vi "Take LTI ULS Reading.vi"(8 "error in (no error)":errorcluster, 11 "MWWL Verification in":refnum<class "MWWL Verification.lvclass">) -> (0 "error out":errorcluster, 3 "MWWL Verification out":refnum<class "MWWL Verification.lvclass">)   [LabVIEW 2017, in "MWWL Verification.lvlib" / "MWWL Verification.lvclass"]
uses:
  MWWL Verification.lvclass
  LTI ULS Actor/LTI ULS Actor Messages/Measure LTI ULS Msg/Measure LTI ULS Msg.lvclass
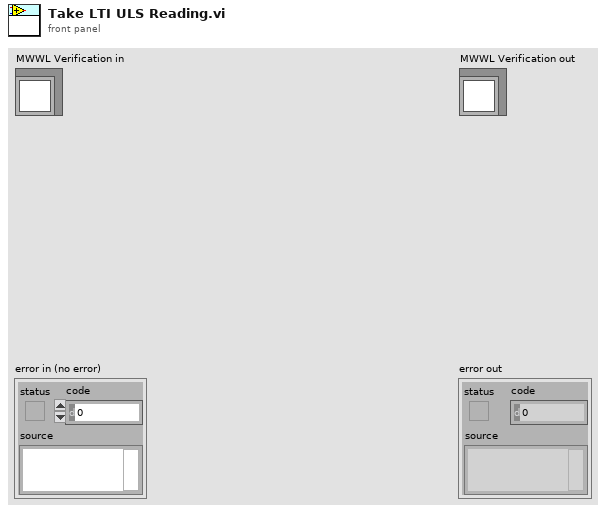
[diagram p1: front panel]
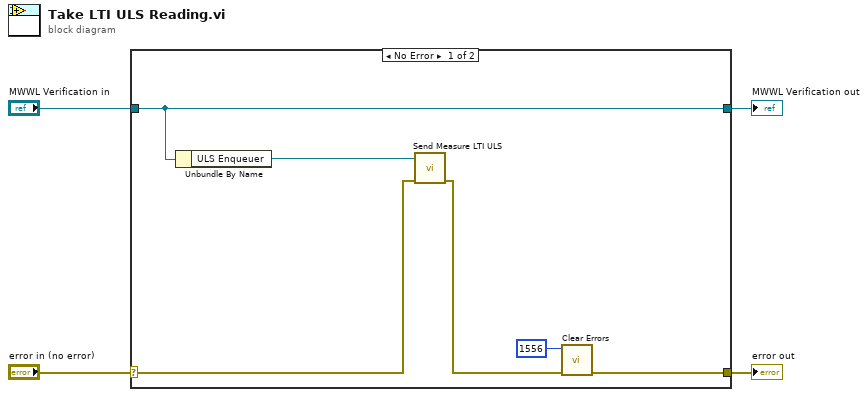
[diagram p0: block diagram]
diagram:
  n1 = case shown="No Error" "error in (no error)" {
    selector: "error in (no error)" -> [w8 w12]
    tunnel: [w5 w12] -> w3
    tunnel: [w10 w11] -> w1
    tunnel: "MWWL Verification in" -> [w10 w11]
    frame No Error {
      n2 = Unbundle By Name(w10) -> ("ULS Enqueuer"=w9:refnum<class "Message Enqueuer.lvclass">)
      n3 = call "Send Measure LTI ULS.vi"("error in (no error)"=w8, "Message Enqueuer in"=w9) -> ("error out"=w6:errorcluster)  [unwired: 8 in, 1 out]
      n4 = call <vilib>:"Clear Errors.vi"("error in (no error)"=w6, "specific error code to clear (0: all)"=1556) -> ("error out"=w5:errorcluster)  [unwired: 4 in, 1 out]
    }
    frame Error {
    }
  }
  "error out" <- w3
  "MWWL Verification out" <- w1
